vi "DHE_ReplaceMacroArgs.vi"(9 "args":string[](array[string]), 10 "command in":string) -> (2 "comand out":string)   [LabVIEW 2016]
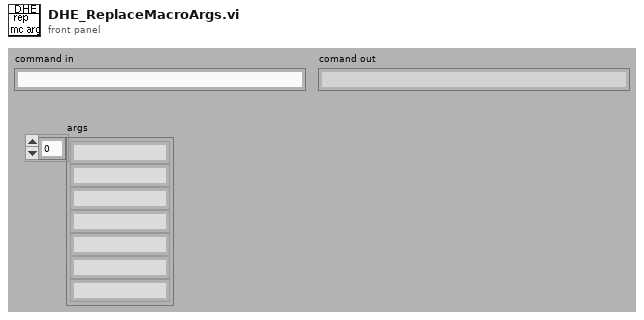
[diagram p1: front panel]
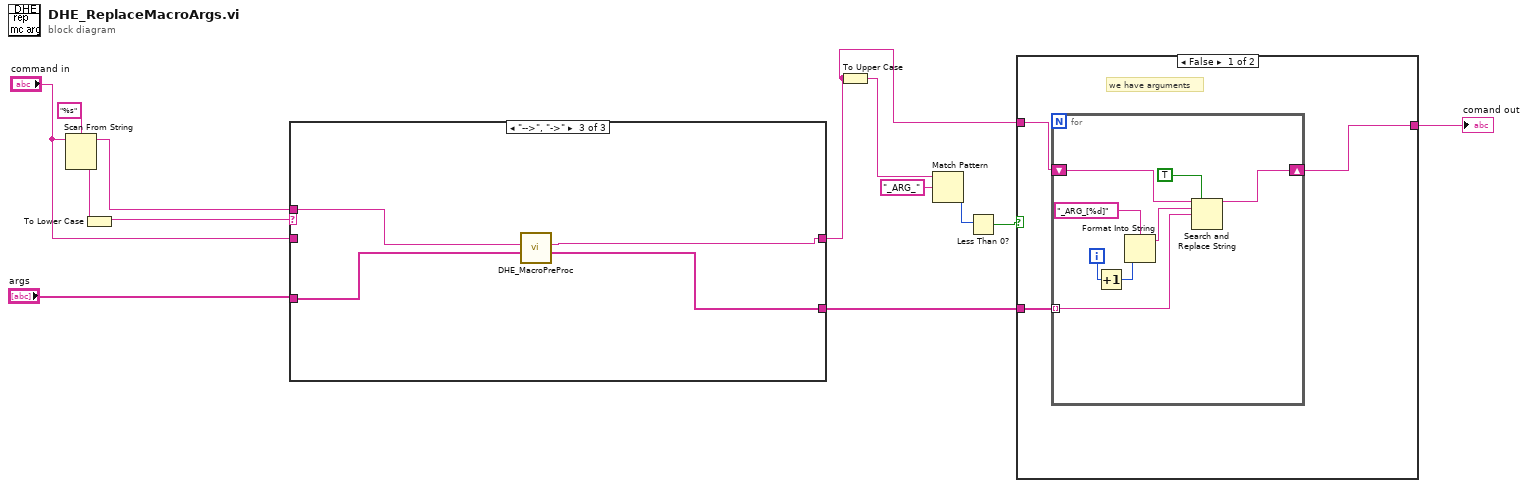
[diagram p0: block diagram]
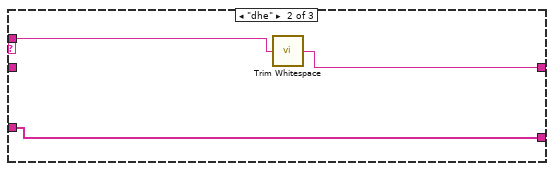
[diagram p3: hidden frame]
diagram:
  n1 = Scan From String(format string="%s", input string="command in") -> (remaining string=w3:string, output 1=w7:string)  [unwired: 2 in, 3 out]
  n2 = To Lower Case(string=w7) -> (all lower case string=w6:string)
  n3 = case shown="\"-->\", \"->\"" w6 {
    tunnel: "command in" -> [w15 _ _]
    tunnel: [w15 w17 w19] -> w4
    tunnel: w3 -> [_ w18 w22]
    tunnel: "args" -> [w14 w16 w21]
    tunnel: [w14 w16 w20] -> w1
    frame Default {
    }
    frame "dhe" {
      n4 = call <vilib>:"Trim Whitespace.vi"("string"=w18) -> ("trimmed string"=w17:string)  [unwired: 1 in]
    }
    frame "-->", "->" {
      n5 = call "DHE_MacroPreProc.vi"("args"=w21, "cmds in"=w22) -> ("args out"=w20:string[], "cmd out"=w19:string)  [unwired: 8 in]
    }
  }
  n6 = To Upper Case(1:w4) -> (0:w10:string)
  n7 = Match Pattern(string=w10, regular expression="_ARG_") -> (offset past match=w11:i32)  [unwired: 4 out]
  n8 = Less Than 0?(x=w11) -> (x < 0?=w9:bool)
  n9 = case shown="False" w9 {
    tunnel: w4 -> [w24 w34]
    tunnel: [w23 w34] -> w13
    tunnel: w1 -> [w25 _]
    frame False {
      # "we have arguments"
      n10 = for {
        tunnel: w25 -> [w31] mode=indexing
        shift-right: [w26] -> w23
        shift-left: w24 -> [w33]
        i -> [w30]
        n11 = Increment(x=w30) -> (x+1=w29:i32)
        n12 = Format Into String(format string="_ARG_[%d]", w29) -> (resulting string=w27:string)  [unwired: 2 in, 1 out]
        n13 = Search and Replace String(replace all?=TRUE ("replace all? (F)"), input string=w33, search string=w27, replace string=w31) -> (result string=w26:string)  [unwired: 1 in, 6 out]
      }
    }
    frame True {
      # "no arguments needed"
    }
  }
  "comand out" <- w13
